vi "Check move conditions.vi"(8 "error in (no error)":errorcluster, 10 "End-stops":cluster{"ES1":bool, "ES2":bool}, 11 "Direction":T1=enum."CW") -> (0 "error out":errorcluster, 2 "String":string, 3 "Move?":bool)   [LabVIEW 2020]
uses:
  Arduino_stepper/Libraries/Arduino stepper/Support/Motor direction -- enum.ctl
  Arduino_stepper/Libraries/Arduino stepper/Arduino stepper.lvlib
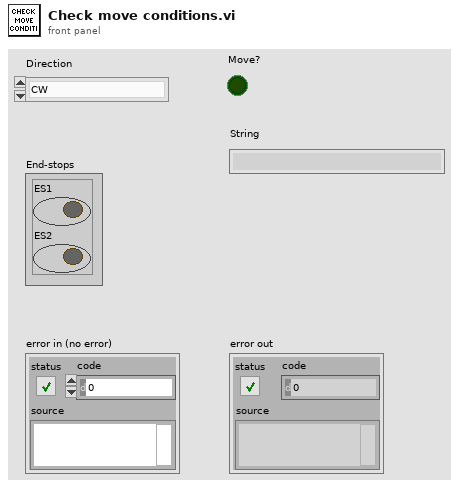
[diagram p1: front panel]
types:
  T1 = typedef "Arduino stepper.lvlib/Motor direction -- enum.ctl" = enum8{"", "CW", "CCW"}
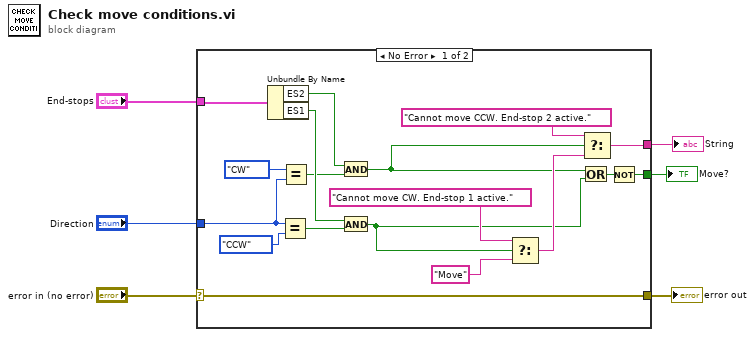
[diagram p0: block diagram]
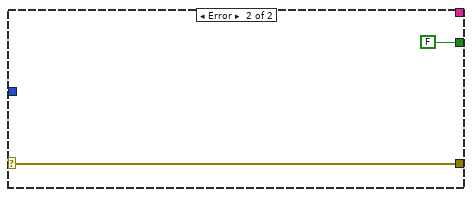
[diagram p2: hidden frame]
diagram:
  n1 = case shown="No Error" "error in (no error)" {
    selector: "error in (no error)" -> [w23 w26]
    tunnel: [w23 w26] -> w5
    tunnel: [w7 FALSE] -> w4
    tunnel: "End-stops" -> [w24 _]
    tunnel: "Direction" -> [w19 _]
    tunnel: [w11 _] -> w1
    frame No Error {
      n2 = Unbundle By Name(w24) -> ("ES2"=w16:bool, "ES1"=w20:bool)
      n3 = Equal?(x=w19, y=enum8{"", "CW", "CCW"}."CCW") -> (x = y?=w21:bool)
      n4 = Equal?(x=enum8{"", "CW", "CCW"}."CW", y=w19) -> (x = y?=w17:bool)
      n5 = And(x=w16, y=w17) -> (x .and. y?=w10:bool)
      n6 = And(x=w20, y=w21) -> (x .and. y?=w9:bool)
      n7 = Select(t="Cannot move CW. End-stop 1 active.", s=w9, f="Move") -> (s? t:f=w12:string)
      n8 = Or(x=w10, y=w9) -> (x .or. y?=w8:bool)
      n9 = Select(t="Cannot move CCW. End-stop 2 active.", s=w10, f=w12) -> (s? t:f=w11:string)
      n10 = Not(x=w8) -> (.not. x?=w7:bool)
    }
    frame Error {
    }
  }
  "error out" <- w5
  "Move?" <- w4
  "String" <- w1
